vi "Leaderboard test.vi"() -> ()   [LabVIEW 2020, in "Visualisation.lvclass"]
uses:
  Visualisation.lvclass
  Application/Globals.vi
  Data Manager/Data Manager.lvclass
  Application/Application.lvlib
panel:
  out "Leaderboard":T1(array[cluster]) {"Distance" scale=0.0..48.9661}
  out "B Total":dbl format="%0.1f km"
  out "A Total":dbl format="%0.1f km"
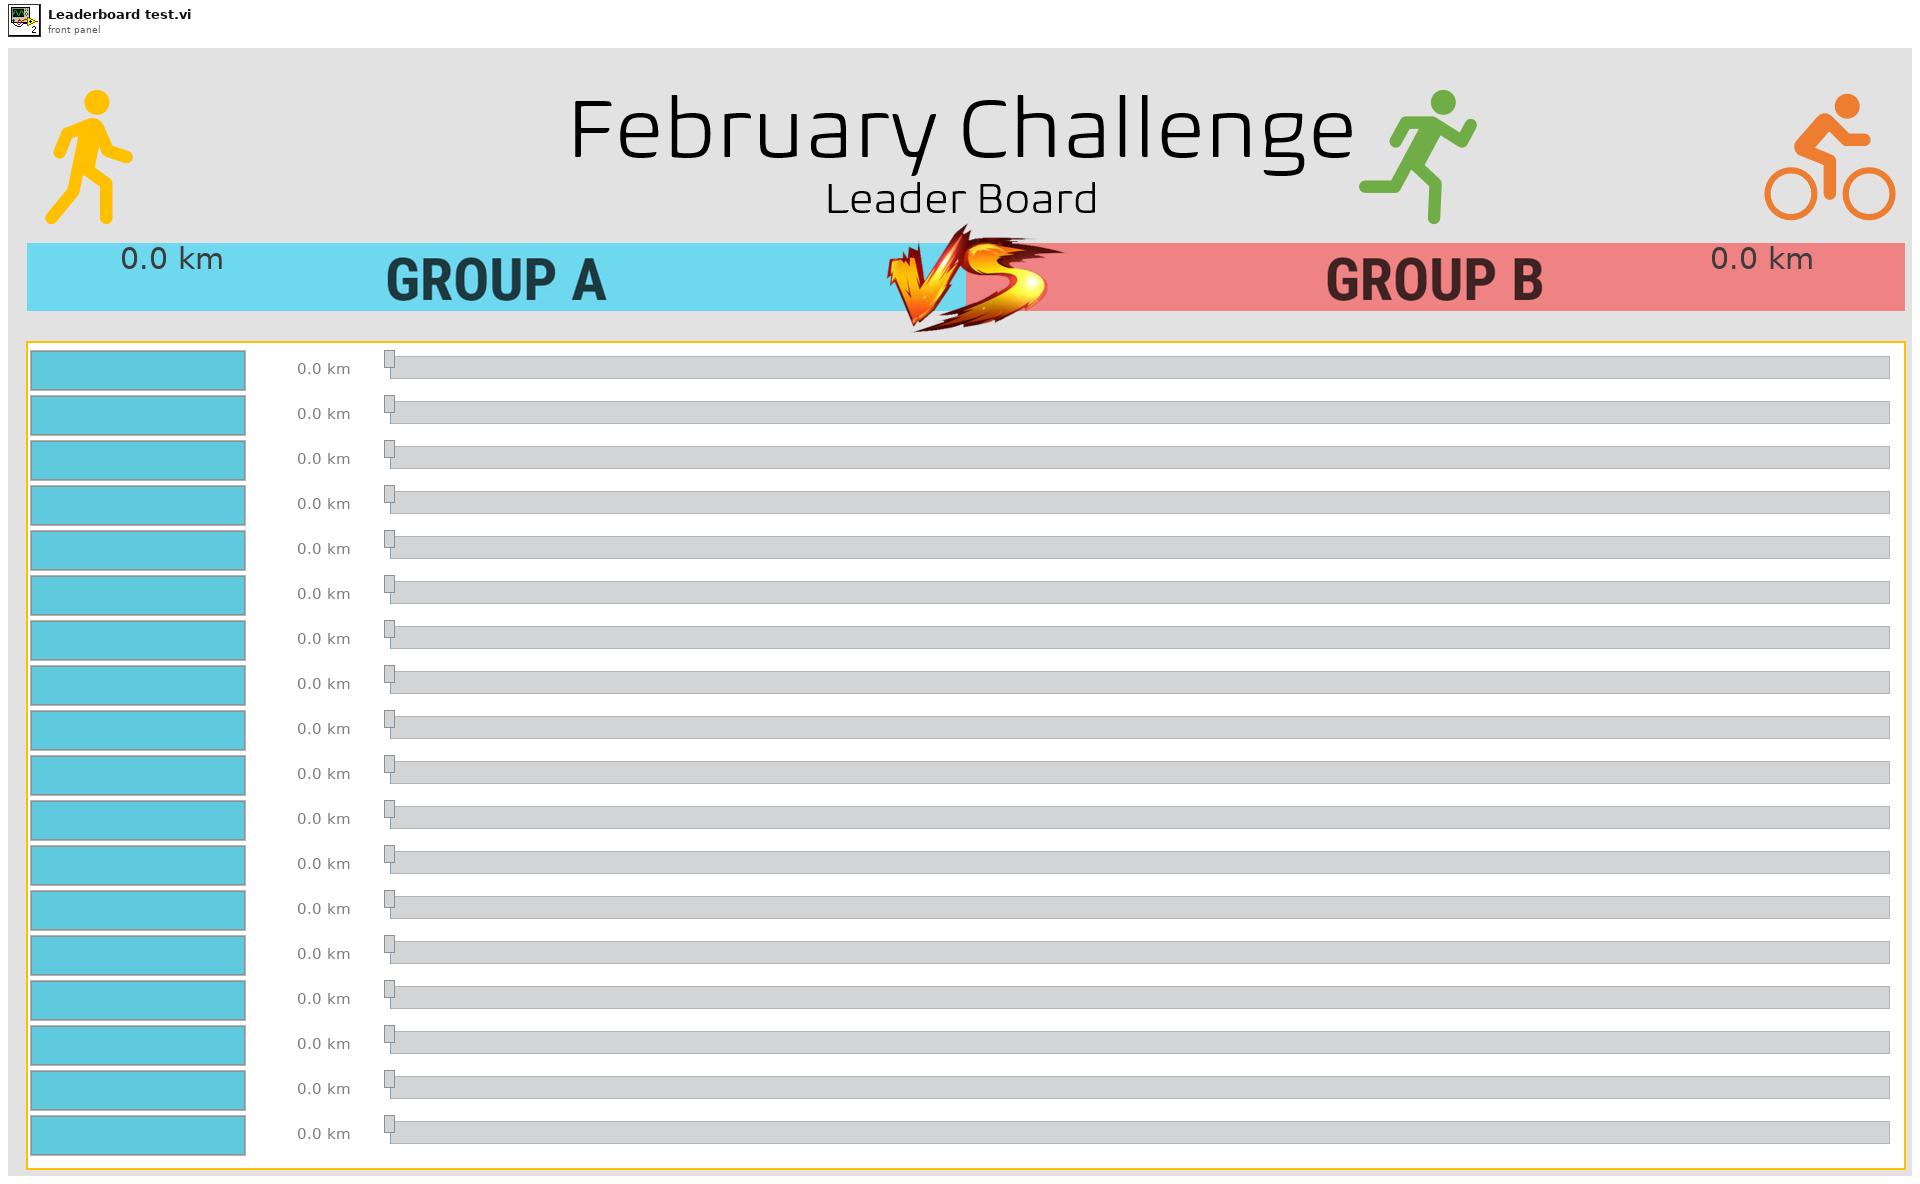
[diagram p1: front panel]
types:
  T1 = cluster{"Athlete":string, "Distance":dbl, "Team":u32}[]
  T2 = cluster{"Athlete":string, "Distance":dbl, "Team":u32}
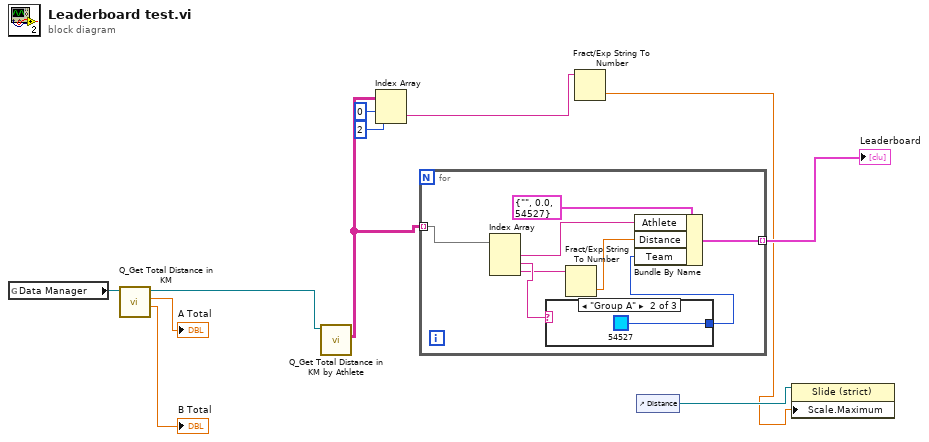
[diagram p0: block diagram]
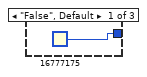
[diagram p2: hidden frame]
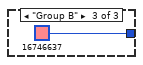
[diagram p3: hidden frame]
diagram:
  n1 = global read "Globals.vi" "Data Manager"() -> (w11:refnum<class "Data Manager.lvclass">)
  n2 = call-dynamic "Q_Get Total Distance in KM.vi"("Data Manager in"=w11) -> ("Group B"=→"B Total":dbl, "Group A"=→"A Total":dbl, "Data Manager out"=w8:refnum<class "Data Manager.lvclass">)  [unwired: 6 in, 2 out]
  n3 = call-dynamic "Q_Get Total Distance in KM by Athlete.vi"("Data Manager in"=w8) -> ("Result Set"=w1:string[][])  [unwired: 8 in, 2 out]
  n4 = Index Array(array=w1, index (row)=0, index (col)=2 ("disabled index (col)")) -> (element=w3:string)
  n5 = for {
    tunnel: w1 -> [w17] mode=indexing
    tunnel: [w18] -> w4 mode=indexing
    n6 = Index Array(array=w17) -> (element #1=w16:string, element #2=w13:string, element #3=w12:string)  [unwired: 3 in]
    n7 = case shown="\"Group A\"" w13 {
      tunnel: [u32 16777175 ("Color Box") u32 54527 ("Color Box") u32 16746637 ("Color Box")] -> w14
      frame "False", Default {
      }
      frame "Group A" {
      }
      frame "Group B" {
      }
    }
    n8 = Fract/Exp String To Number(string=w12) -> (number=w15:dbl)  [unwired: 3 in, 1 out]
    n9 = Bundle By Name(cluster=T2 {"Athlete"="", "Distance"=0.0, "Team"=54527} ("Leaderboard"), "Athlete"=w16, "Distance"=w15, "Team"=w14) -> (w18:T2)
  }
  "Leaderboard" <- w4
  n10 = Fract/Exp String To Number(string=w3) -> (number=w2:dbl)  [unwired: 3 in, 1 out]
  n11 = control-ref of="Distance"() -> (w7:refnum<vi>)
  n12 = property on="Property Node" class="Slide (strict)"(reference=w7, "Scale.Maximum"=w2) -> ()  [unwired: 1 in, 2 out]
